vi "Init and Rotate array UInt32.vi"(5 "Reset":bool, 7 "Stop read":bool, 9 "Array size":i32=30, 11 "PV":u32) -> (3 "Array":u32[](array[numeric]))   [LabVIEW 2019, in "Userlib.lvlib"]
uses:
  Userlib.lvlib
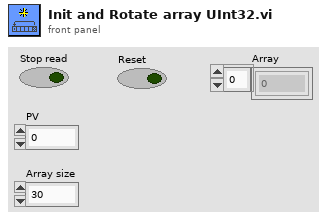
[diagram p1: front panel]
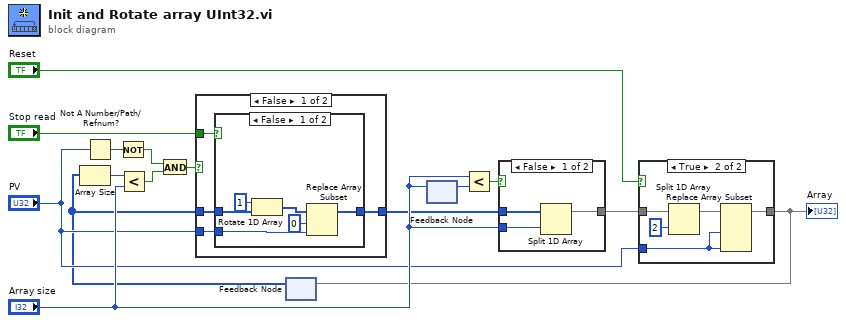
[diagram p0: block diagram]
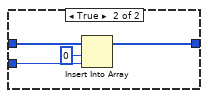
[diagram p3: hidden frame]
diagram:
  n1 = Not A Number/Path/Refnum?(number/path/refnum="PV") -> (NaN/Path/Refnum?=w13:bool)
  n2 = Not(x=w13) -> (.not. x?=w12:bool)
  n3 = feedback #1() -> (w1:u32[])  [unwired: 1 in]
  n4 = Array Size(array=w1) -> (size(s)=w15:i32)
  n5 = Less?(x=w15, y="Array size") -> (x < y?=w14:bool)
  n6 = And(x=w12, y=w14) -> (x .and. y?=w5:bool)
  n7 = case shown="False" w5 {
    tunnel: [w17 w30] -> w4
    tunnel: "PV" -> [w18 w27]
    tunnel: w1 -> [w19 w29]
    tunnel: "Stop read" -> [w16 _]
    frame False {
      n8 = case shown="False" w16 {
        tunnel: w19 -> [w22 w26]
        tunnel: w18 -> [w21 _]
        tunnel: [w20 w26] -> w17
        frame False {
          n9 = Rotate 1D Array(1:w22, 2:1 ("n")) -> (0:w24:u32[])
          n10 = Replace Array Subset(array=w24, new element=w21, index=0) -> (w20:u32[])
        }
        frame True {
        }
      }
    }
    frame True {
      n11 = Insert Into Array(array=w29, index=0, new element=w27) -> (w30:u32[])
    }
  }
  n12 = feedback #2() -> (w11:i32)  [unwired: 1 in]
  n13 = feedback-in #2("Array size") -> ()
  n14 = Less?(x="Array size", y=w11) -> (x < y?=w10:bool)
  n15 = case shown="False" w10 {
    tunnel: [w31 w34] -> w7
    tunnel: w4 -> [w33 w34]
    tunnel: "Array size" -> [w32 _]
    frame False {
      n16 = Split 1D Array(array=w33, index=w32) -> (first subarray=w31:u32[])  [unwired: 1 out]
    }
    frame True {
    }
  }
  n17 = case shown="True" "Reset" {
    tunnel: [w35 w37] -> w6
    tunnel: w7 -> [w35 w40]
    tunnel: "PV" -> [_ w36]
    frame False {
    }
    frame True {
      n18 = Split 1D Array(array=w40, index=2) -> (first subarray=w39:u32[])  [unwired: 1 out]
      n19 = Replace Array Subset(array=w39, new element #1=w36, new element #2=w36) -> (w37:u32[])  [unwired: 2 in]
    }
  }
  "Array" <- w6
  n20 = feedback-in #1(w6) -> ()
